vi "Close.vi"(8 "error in (no error)":errorcluster, 11 "PF_API in":refnum<class "PF_API.lvclass">) -> (0 "error out":errorcluster, 3 "PF_API out":refnum<class "PF_API.lvclass">)   [LabVIEW 2019, in "PF_API.lvclass"]
doc: "Finishes the communication session with the scanner."
uses:
  PF_API.lvclass
  PF_API.lvclass/PF_API.ctl
  <vilib>/httpClient/LabVIEWHTTPClient.lvlib
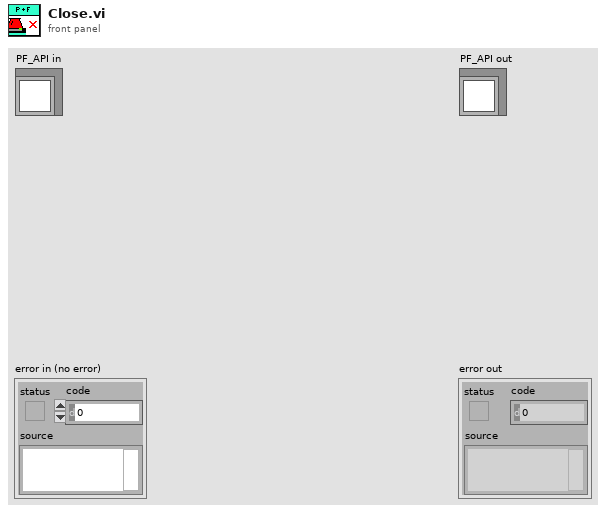
[diagram p1: front panel]
types:
  T1 = typedef "LabVIEWHTTPClient.lvlib/ClientHandle.ctl" = refnum<k1>
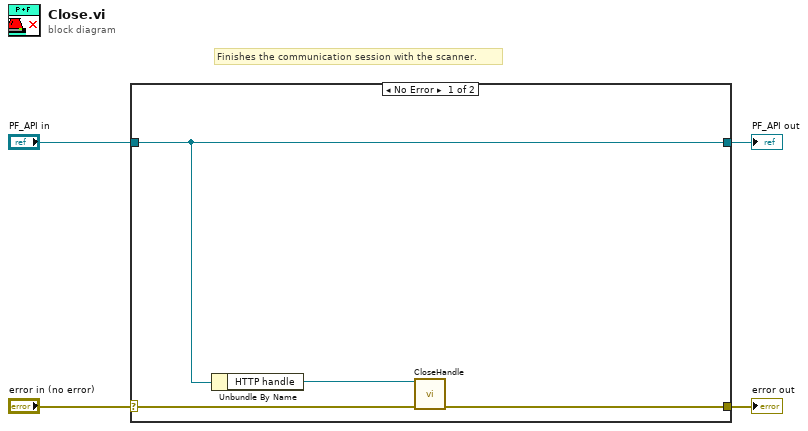
[diagram p0: block diagram]
diagram:
  # "Finishes the communication session with the scanner."
  n1 = case shown="No Error" "error in (no error)" {
    selector: "error in (no error)" -> [w8 w10]
    tunnel: [w7 w10] -> w3
    tunnel: [w6 w9] -> w1
    tunnel: "PF_API in" -> [w6 w9]
    frame No Error {
      n2 = Unbundle By Name(w6) -> ("HTTP handle"=w5:T1)
      n3 = call <vilib>:"CloseHandle.vi"("client handle"=w5, "error in (no error)"=w8) -> ("error out"=w7:errorcluster)  [unwired: 13 in]
    }
    frame Error {
    }
  }
  "error out" <- w3
  "PF_API out" <- w1
